vi "MB Ethernet Transmit.vi"(7 "MBAP Header":T1, 8 "error in (no error)":errorcluster, 9 "Timeout":i32=10000, 10 "Modbus Data Unit":T2={"Function Code"=1, "Data"=[]} {"Function Code" items=["Read Coils"=1, "Read Discrete Inputs"=2, "Read Holding Registers"=3, "Read Input Registers"=4, "Write Single Coil"=5, "Write Single Register"=6, "Read Exception Status"=7, "Write Multiple Coils"=15, "Write Multiple Registers"=16]; "Data" format="%.0x"}, 11 "TCP Connection Refnum in":refnum<k5>) -> (0 "error out":errorcluster, 3 "TCP Connection Refnum (dup)":refnum<k5>)   [LabVIEW 2010]
uses:
  MB Modbus Data Unit.ctl
panel:
  # "VI Name: MB Serial Transmit.vi\nPurpose: Sends a Modbus message.\nReentrant because its caller is reentrant."
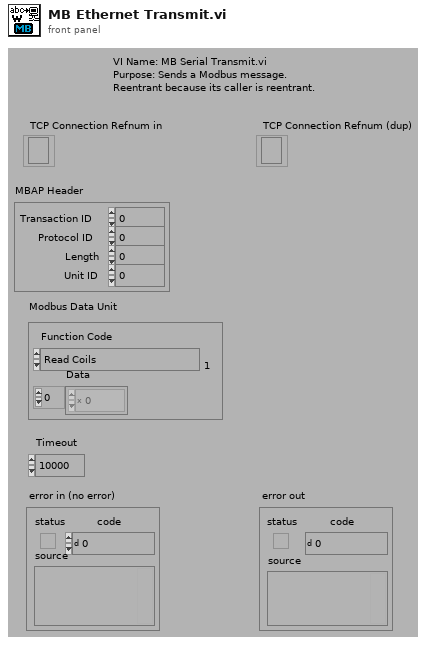
[diagram p1: front panel]
types:
  T1 = cluster{"Transaction ID":u16, "Protocol ID":u16, "Length":u16, "Unit ID":u8}
  T2 = typedef "MB Modbus Data Unit.ctl" = cluster{"Function Code":u8, "Data":u8[]}
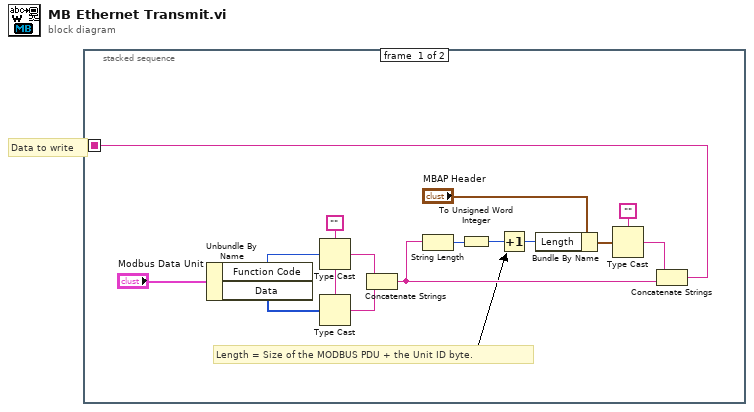
[diagram p0: block diagram]
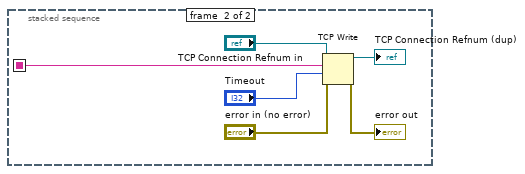
[diagram p2: hidden frame]
diagram:
  # "Data to write"
  n1 = stacked-sequence {
    seq-local: [w2 _] -> [_ w21]
    frame #0 {
      w15 = ""
      # "Length = Size of the MODBUS PDU + the Unit ID byte."
      n2 = Unbundle By Name("Modbus Data Unit") -> ("Function Code"=w11:u8, "Data"=w10:u8[])
      n3 = Type Cast(type=w15, x=w11) -> (*(type *) &x=w14:string)
      n4 = Type Cast(type=w15, x=w10) -> (*(type *) &x=w13:string)
      n5 = Concatenate Strings(w14, w13) -> (w3:string)
      n6 = String Length(string=w3) -> (length=w8:i32)
      n7 = To Unsigned Word Integer(number=w8) -> (unsigned 16bit integer=w7:u16)
      n8 = Increment(x=w7) -> (x+1=w1:u16)
      n9 = Bundle By Name(cluster="MBAP Header", "Length"=w1) -> (w5:T1)
      n10 = Type Cast(type="", x=w5) -> (*(type *) &x=w4:string)
      n11 = Concatenate Strings(w4, w3) -> (w2:string)
    }
    frame #1 {
      n12 = TCP Write(connection ID="TCP Connection Refnum in", data in=w21, error in (no error)="error in (no error)", 9:"Timeout") -> (connection ID out=→"TCP Connection Refnum (dup)":refnum<k5>, error out=→"error out":errorcluster)  [unwired: 1 out]
    }
  }
